vi "setup Encoder LV.vi"(0 "filterDepth":u8, 4 "index":u8, 6 "ABS":u8, 8 "resolution":u16, 9 "pinLocation":u8, 10 "encoderNum":u8, 11 "instance":i32) -> (3 "function return":u32)   [LabVIEW 2025, in "SADI_FW3.lvlib"]
doc: "SADI_API_Wrapper unsigned int setupEncoder_LV( int instance ,\n uint8_t encoderNum ,\n uint8_t pinLocation ,\n uint8_t index ,\n uint8_t ABS ,\n uint8_t filterDepth ,\n uint16_t resolution );\nSADI_API_Wrapper unsigned int setupEncoder_LV( int instance ,\n uint8_t encoderNum ,\n uint8_t pinLocation ,\n uint8_t index ,\n uint8_t ABS ,\n uint8_t filterDepth ,\n uint16_t resolution );"
uses:
  SADI_FW3.lvlib
  SADI_FW3.dll
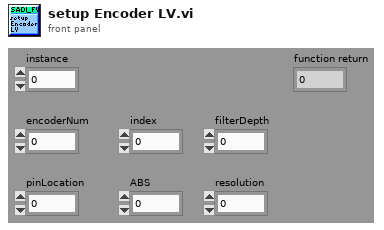
[diagram p1: front panel]
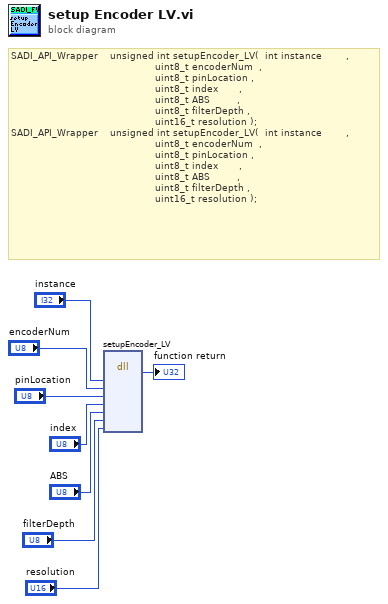
[diagram p0: block diagram]
diagram:
  # "SADI_API_Wrapper    unsigned int setupEncoder_LV(  int instance        ,\n                                                uint8_t encoderNum  ,\n                                                uint8_t pinLocation ,\n                                                uint8_t index       ,\n                                                uint8_t ABS         ,\n                                                uint8_t filterDepth ,\n                                                uint16_t resolution );\nSADI_API_Wrapper    unsigned int setupEncoder_LV(  int instance        ,\n                                                uint8_t encoderNum  ,\n                                                uint8_t pinLocation ,\n                                                uint8_t index       ,\n                                                uint8_t\tABS         ,\n                                                uint8_t\tfilterDepth ,\n                                                uint16_t resolution );"
  n1 = dll-call lib="C:/Users/noaht/School/Fall 2025/Controls Lab/Lab 3/EML4314c_FA25_framework_0/LVLib/SADI_FW3.*" fn="setupEncoder_LV"("instance"="instance", "encoderNum"="encoderNum", "pinLocation"="pinLocation", "index"="index", "ABS"="ABS", "filterDepth"="filterDepth", "resolution"="resolution") -> (→"function return":u32)  [unwired: 10 in, 2 out]
